vi "Abort Movement.vi"(8 "error in (no error)":errorcluster, 11 "CS++Motor in":refnum<class "CS++Motor.lvclass">) -> (0 "error out":errorcluster, 3 "CS++Motor out":refnum<class "CS++Motor.lvclass">)   [LabVIEW 2015, in "CS++Motor.lvlib" / "CS++Motor.lvclass"]
uses:
  CS++Motor.lvclass
  CS++Motor.lvclass/CS++Motor.ctl
  PV-Enum-n.ctl
  CSPP_Core/Classes/CS++ProcessVariables/ProcessVariable/PV.lvclass
  CSPP_Core/Classes/CS++ProcessVariables/ProcessVariable/PV.lvclass/PV.ctl
  CSPP_Core/Classes/CS++ProcessVariables/ProcessVariable/Write Data.vi
  CSPP_Core/Classes/CS++ProcessVariables/ProcessVariable/Write Timestamp.vi
  CSPP_Core/Classes/CS++ProcessVariables/ProcessVariable/Write Quality.vi
  CSPP_Core/Classes/CS++ProcessVariables/ProcessVariable/Write status.vi
  CSPP_Core/Classes/CS++ProcessVariables/PVConnection/PVConnection.lvclass
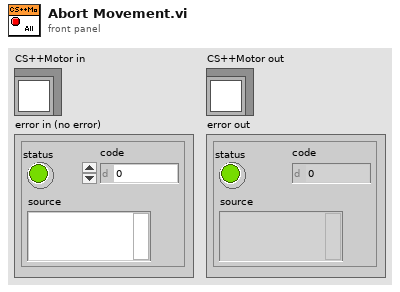
[diagram p1: front panel]
types:
  T1 = typedef "CS++Motor.lvlib/CS++Motor.lvclass/PV-Enum-n.ctl" = enum16{"PhysicalName", "unit", "ActPosition", "SetPosition", "RawSetPosition", "StartVelocity", "StopVelocity", "Acceleration", "RangeMin", "RangeMax", "Scaling", "RangeRefError", "LogicalPositionArray", "NoOfCommands"}
  T2 = cluster{"LogicalName":string, "PhysicalName":string, "unit":string, "Scaling":dbl, "StartVelocity":dbl, "StopVelocity":dbl, "Acceleration":dbl, "RangeMin":dbl, "RangeMax":dbl, "LogicalPos-Array":cluster{"LogicalPosition":string, "SetPosition":dbl}[]}[]
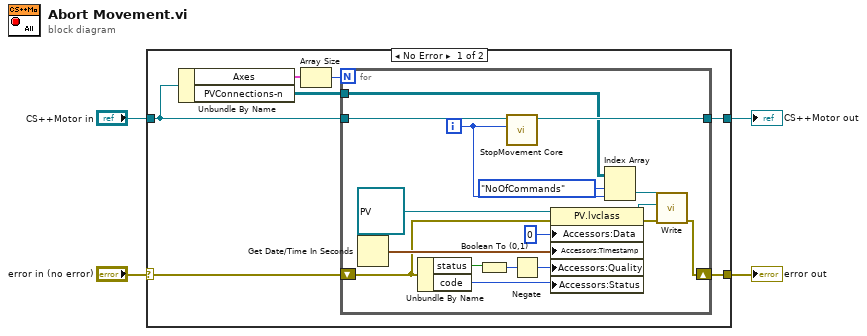
[diagram p0: block diagram]
diagram:
  n1 = case shown="No Error" "error in (no error)" {
    selector: "error in (no error)" -> [w6 w30]
    tunnel: [w5 w30] -> w3
    tunnel: [w10 w29] -> w1
    tunnel: "CS++Motor in" -> [w11 w29]
    frame No Error {
      n2 = Unbundle By Name(w11) -> ("Axes"=w9:T2, "PVConnections-n"=w7:refnum<class "PVConnection.lvclass">[][])
      n3 = Array Size(array=w9) -> (size(s)=w8:i32)
      n4 = for {
        N: w8 -> [_]
        tunnel: w11 -> [w28]
        tunnel: [w27] -> w10
        tunnel: w7 -> [w18]
        shift-right: [w14] -> w5
        shift-left: w6 -> [w15]
        i -> [w13]
        n5 = Get Date/Time In Seconds() -> (seconds since 1Jan1904=w17:timestamp)
        n6 = Unbundle By Name(w15) -> ("status"=w24:bool, "code"=w21:i32)
        n7 = Boolean To (0,1)(Boolean=w24) -> (0, 1=w20:i16)
        n8 = call-dynamic "StopMovement Core.vi"("AxisNumber"=w13, "CS++Motor in"=w28) -> ("CS++Motor out"=w27:refnum<class "CS++Motor.lvclass">)  [unwired: 8 in, 1 out]
        n9 = Negate(x=w20) -> (-x=w25:i16)
        n10 = property class="PV.lvclass"(reference=refnum<class "PV.lvclass"> refnum ("PV"), error in=w15, "Accessors:Data"=0, "Accessors:Timestamp"=w17, "Accessors:Quality"=w25, "Accessors:Status"=w21) -> (reference out=w23:refnum<class "PV.lvclass">, error out=w22:errorcluster)
        n11 = Index Array(array=w18, index (row)=PV-Enum-n."NoOfCommands" ("PV-Enum-n"), index (col)=w13) -> (element=w19:refnum<class "PVConnection.lvclass">)
        n12 = call "Write.vi"("error in (no error)"=w22, "PV"=w23, "PVConnection in"=w19) -> ("error out"=w14:errorcluster)  [unwired: 7 in, 1 out]
      }
    }
    frame Error {
    }
  }
  "error out" <- w3
  "CS++Motor out" <- w1
